vi "HardwareLoop.vi"(8 "Error In":errorcluster, 10 "Action Queues":T2, 11 "Executable Configuration":T1) -> (0 "Error Out":errorcluster)   [LabVIEW 2012]
uses:
  ActionQueues.ctl
  UIActionQueueElement.ctl
  UIAction.ctl
  HardwareActionQueueElement.ctl
  HardwareAction.ctl
  ExecutableConfiguration.ctl
  driver/Keithley-7001.lvlib
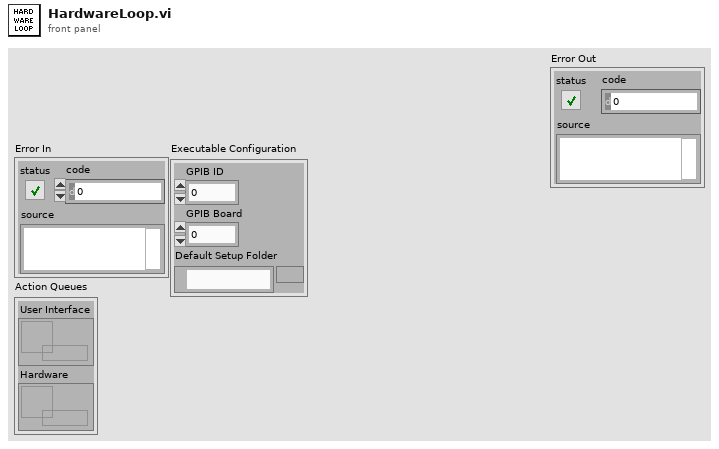
[diagram p1: front panel]
types:
  T1 = typedef "ExecutableConfiguration.ctl" = cluster{"GPIB ID":u8, "GPIB Board":u8, "Default Setup Folder":path}
  T2 = typedef "ActionQueues.ctl" = cluster{"User Interface":refnum<queue>, "Hardware":refnum<queue>}
  T3 = typedef "HardwareActionQueueElement.ctl" = cluster{"Action":T4, "Data":variant}
  T4 = typedef "HardwareAction.ctl" = enum16{"Initialize", "Start", "Stop", "Error", "Shutdown"}
  T5 = typedef "UIActionQueueElement.ctl" = cluster{"Action":T6, "Data":variant}
  T6 = typedef "UIAction.ctl" = enum16{"Initialize", "Configure Trigger", "Configure Scan", "Configure Memory", "Configure Slot 1", "Open", "Save", "Reset", "Start", "Started", "Stop", "Stopped", "Shutdown"}
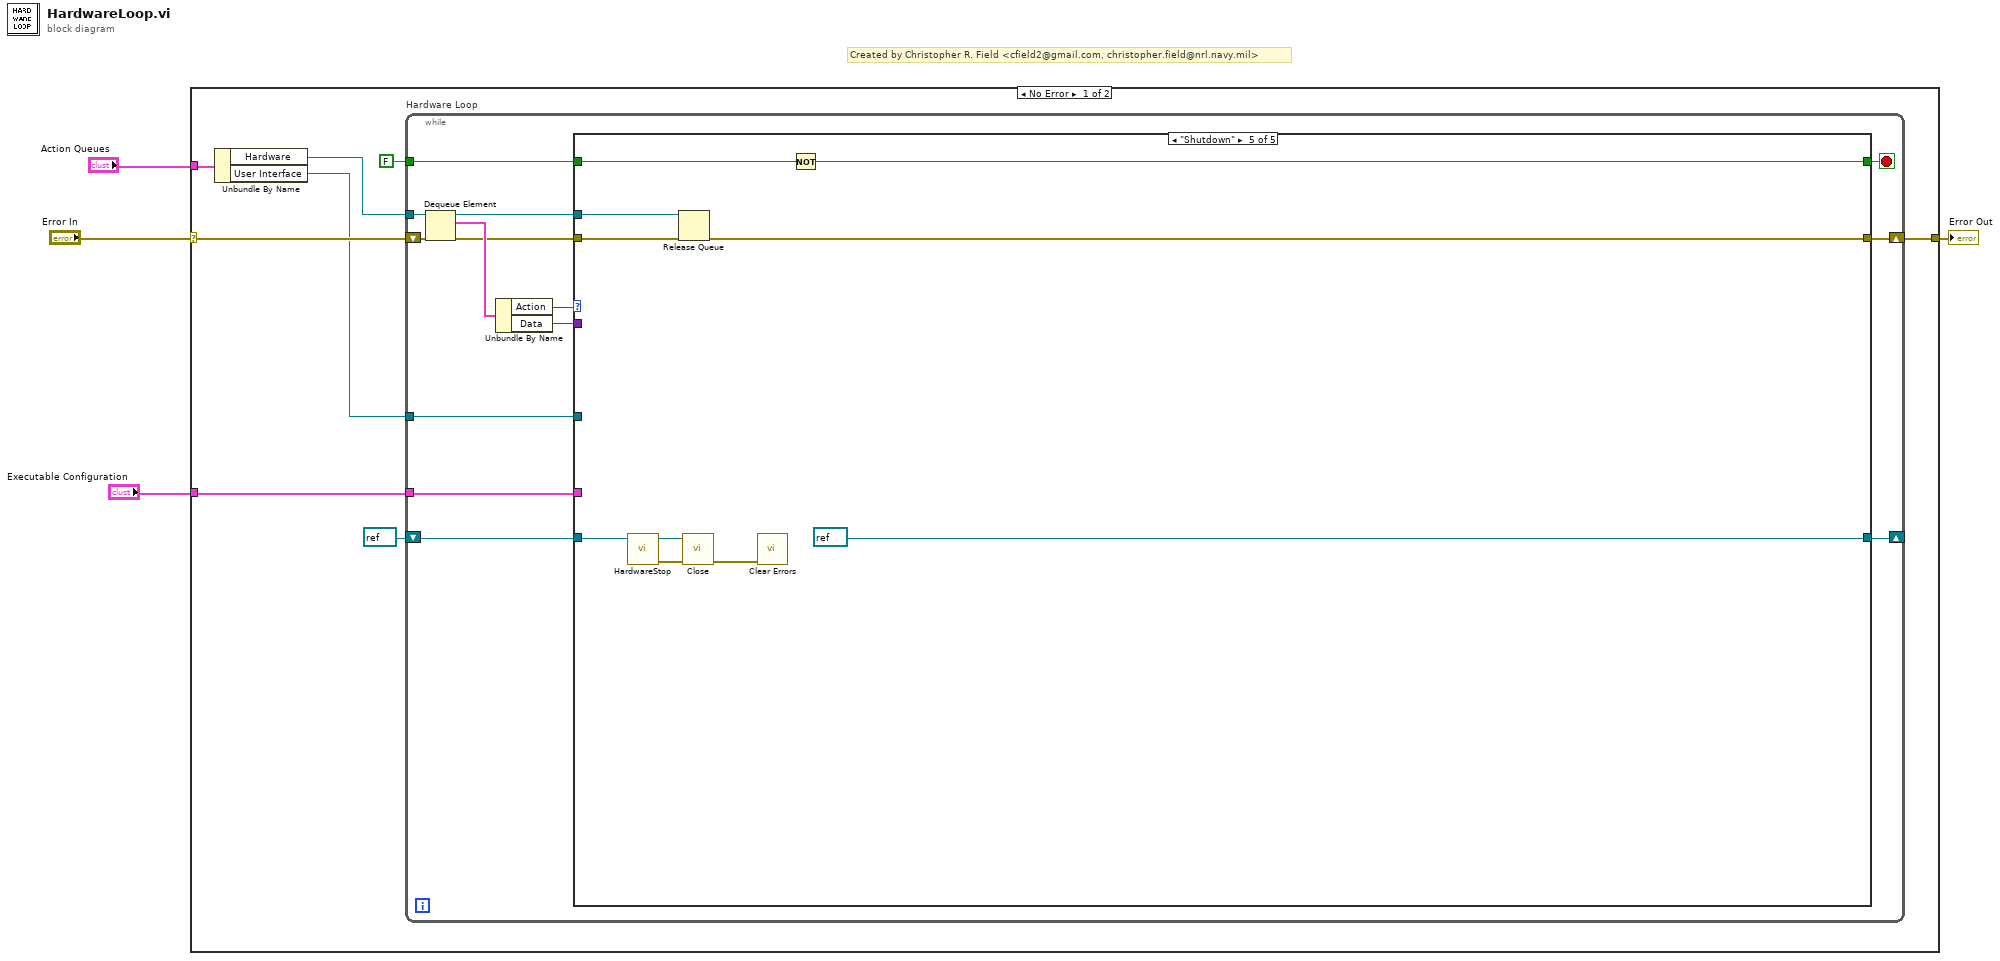
[diagram p0: block diagram]
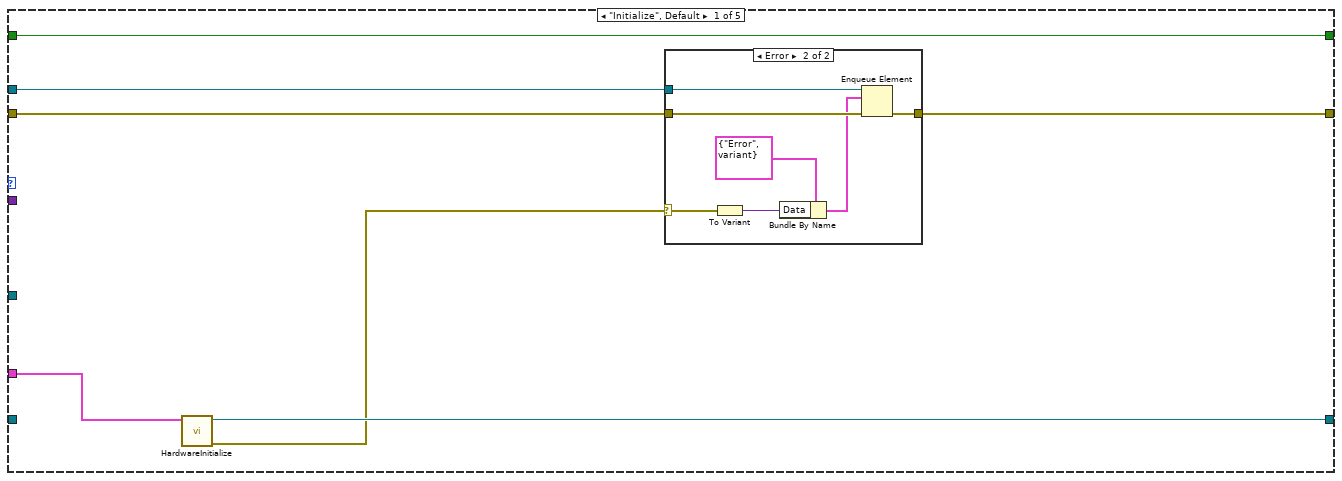
[diagram p2: hidden frame]
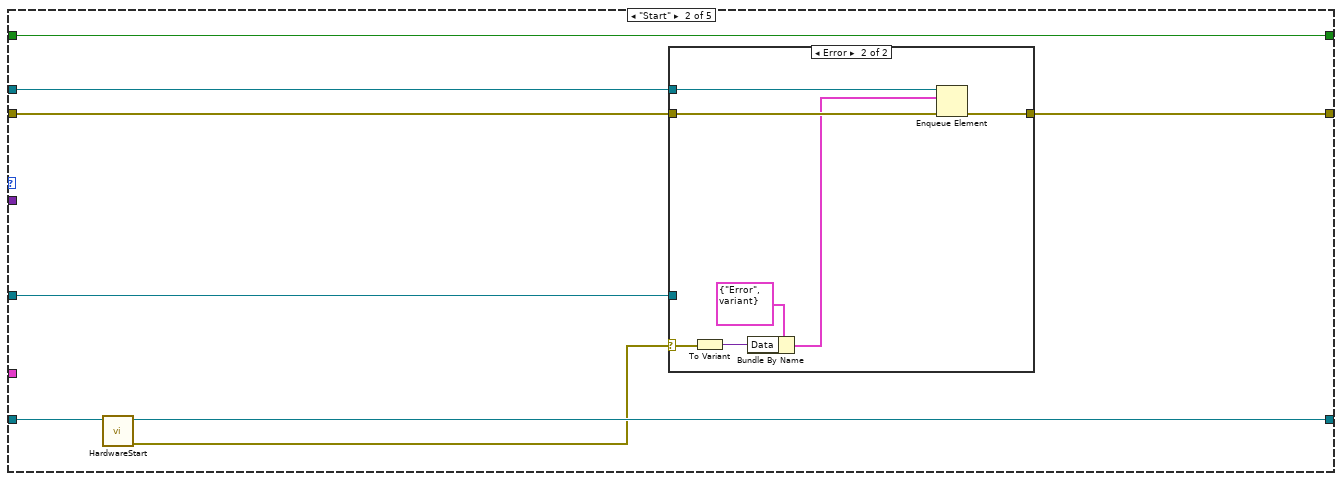
[diagram p4: hidden frame]
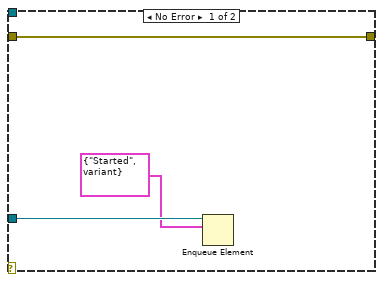
[diagram p5: hidden frame]
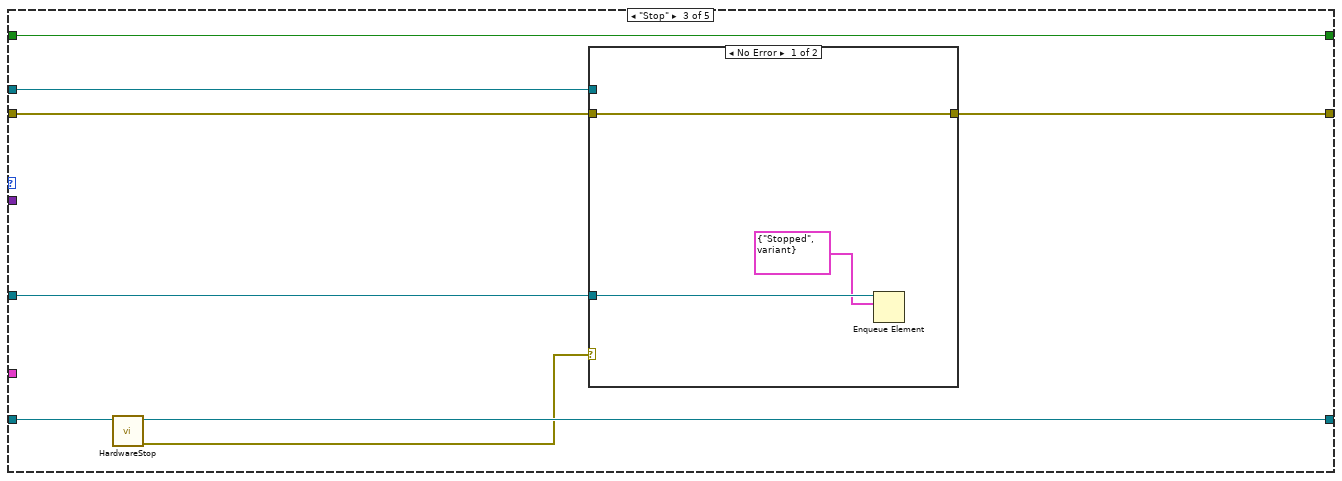
[diagram p6: hidden frame]
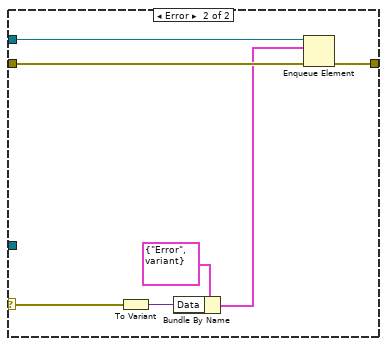
[diagram p7: hidden frame]
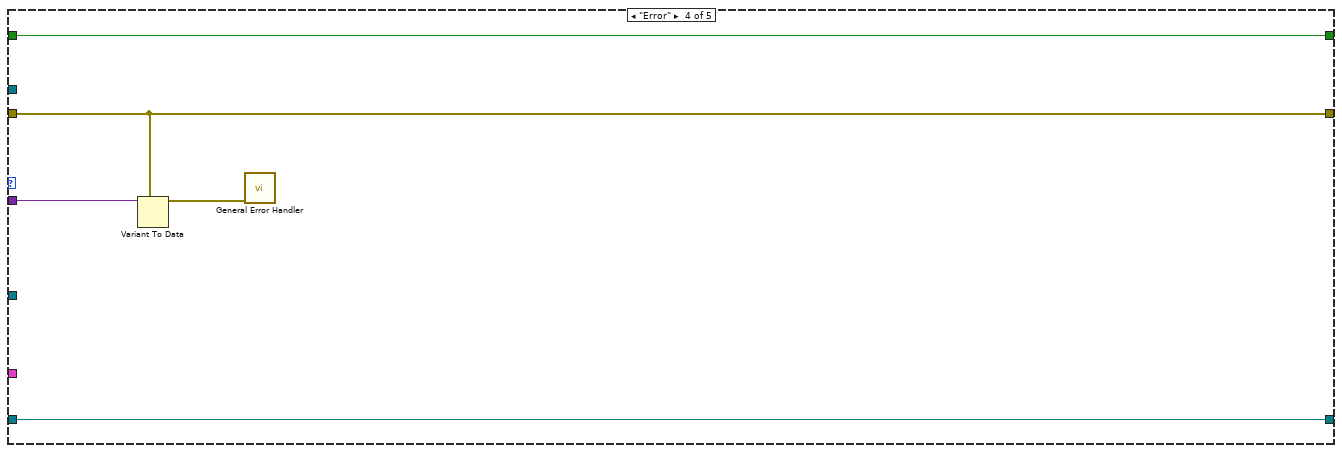
[diagram p8: hidden frame]
diagram:
  # "Created by Christopher R. Field <cfield2@gmail.com, christopher.field@nrl.navy.mil>"
  n1 = case shown="No Error" "Error In" {
    selector: "Error In" -> [w12 w93]
    tunnel: "Action Queues" -> [w11 _]
    tunnel: "Executable Configuration" -> [w7 _]
    tunnel: [w6 w93] -> w1
    frame No Error {
      n2 = Unbundle By Name(w11) -> ("Hardware"=w10:refnum<queue>, "User Interface"=w8:refnum<queue>)
      n3 = while "Hardware Loop" {
        tunnel: w10 -> [w25]
        shift-right: [w17] -> w6
        shift-left: w12 -> [w26]
        tunnel: FALSE -> [w19]
        tunnel: w8 -> [w16]
        tunnel: w7 -> [w15]
        shift-right: [w14] -> _
        shift-left: refnum<visa-resource-name> refnum ("Keithley 7001 Out") -> [w13]
        stop <- w18 stop-if-true
        n4 = Dequeue Element(queue=w25, error in (no error)=w26) -> (queue out=w20:refnum<queue>, element=w24:T3, error out=w21:errorcluster)  [unwired: 1 in, 1 out]
        n5 = Unbundle By Name(w24) -> ("Action"=w23:T4, "Data"=w22:variant)
        n6 = case shown="\"Shutdown\"" w23 {
          tunnel: w22 -> [_ _ _ w81 _]
          tunnel: w21 -> [w32 w44 w60 w80 w89]
          tunnel: w20 -> [w30 w45 w61 _ w90]
          tunnel: w19 -> [w33 w49 w67 w82 w92]
          tunnel: [w33 w49 w67 w82 w91] -> w18
          tunnel: [w31 w43 w64 w80 w88] -> w17
          tunnel: w16 -> [_ w42 w62 _ _]
          tunnel: w15 -> [w28 _ _ _ _]
          tunnel: [w29 w47 w65 w78 refnum<visa-resource-name> refnum ("Keithley 7001 Out")] -> w14
          tunnel: w13 -> [_ w48 w66 w78 w83]
          frame "Initialize", Default {
            n7 = call "HardwareInitialize.vi"("Executable Configuration"=w28) -> ("Error Out"=w27:errorcluster, "Keithley 7001 Out"=w29:refnum<visa-resource-name>)  [unwired: 9 in]
            n8 = case shown="Error" w27 {
              selector: w27 -> [_ w36]
              tunnel: w32 -> [w34 w41]
              tunnel: [w34 w40] -> w31
              tunnel: w30 -> [_ w39]
              frame No Error {
              }
              frame Error {
                n9 = To Variant(anything=w36) -> (Variant=w37:variant)
                n10 = Bundle By Name(cluster=T3 {"Action"=enum."Error", "Data"=variant} ("element"), "Data"=w37) -> (w35:T3)
                n11 = Enqueue Element(queue=w39, element=w35, error in (no error)=w41) -> (error out=w40:errorcluster)  [unwired: 1 in, 2 out]
              }
            }
          }
          frame "Start" {
            n12 = call "HardwareStart.vi"("Keithley 7001 In"=w48) -> ("Error Out"=w46:errorcluster, "Keithley 7001 Out"=w47:refnum<visa-resource-name>)  [unwired: 9 in]
            n13 = case shown="Error" w46 {
              selector: w46 -> [_ w54]
              tunnel: w45 -> [_ w59]
              tunnel: w44 -> [w52 w58]
              tunnel: [w52 w57] -> w43
              tunnel: w42 -> [w51 _]
              frame No Error {
                n14 = Enqueue Element(queue=w51, element=T5 {"Action"=enum."Started", "Data"=variant}) -> ()  [unwired: 2 in, 3 out]
              }
              frame Error {
                n15 = To Variant(anything=w54) -> (Variant=w55:variant)
                n16 = Bundle By Name(cluster=T3 {"Action"=enum."Error", "Data"=variant} ("element"), "Data"=w55) -> (w53:T3)
                n17 = Enqueue Element(queue=w59, element=w53, error in (no error)=w58) -> (error out=w57:errorcluster)  [unwired: 1 in, 2 out]
              }
            }
          }
          frame "Stop" {
            n18 = call "HardwareStop.vi"("Keithley 7001 In"=w66) -> ("Error Out"=w63:errorcluster, "Keithley 7001 Out"=w65:refnum<visa-resource-name>)  [unwired: 9 in]
            n19 = case shown="No Error" w63 {
              selector: w63 -> [_ w72]
              tunnel: w61 -> [_ w77]
              tunnel: w60 -> [w70 w76]
              tunnel: [w70 w75] -> w64
              tunnel: w62 -> [w69 _]
              frame No Error {
                n20 = Enqueue Element(queue=w69, element=T5 {"Action"=enum."Stopped", "Data"=variant}) -> ()  [unwired: 2 in, 3 out]
              }
              frame Error {
                n21 = To Variant(anything=w72) -> (Variant=w73:variant)
                n22 = Bundle By Name(cluster=T3 {"Action"=enum."Error", "Data"=variant} ("element"), "Data"=w73) -> (w71:T3)
                n23 = Enqueue Element(queue=w77, element=w71, error in (no error)=w76) -> (error out=w75:errorcluster)  [unwired: 1 in, 2 out]
              }
            }
          }
          frame "Error" {
            n24 = Variant To Data(type=w80, Variant=w81) -> (data=w79:errorcluster)  [unwired: 1 in, 1 out]
            n25 = call <vilib>:"General Error Handler.vi"("error in (no error)"=w79) -> ()  [unwired: 10 in, 5 out]
          }
          frame "Shutdown" {
            n26 = call "HardwareStop.vi"("Keithley 7001 In"=w83) -> ("Error Out"=w85:errorcluster, "Keithley 7001 Out"=w84:refnum<visa-resource-name>)  [unwired: 9 in]
            n27 = Release Queue(queue=w90, error in (no error)=w89) -> (error out=w88:errorcluster)  [unwired: 1 in, 2 out]
            n28 = call "Close.vi"("Error In"=w85, "Keithley 7001 In"=w84) -> ("Error Out"=w87:errorcluster)  [unwired: 9 in]
            n29 = call <vilib>:"Clear Errors.vi"("error in (no error)"=w87) -> ()  [unwired: 6 in, 1 out]
            n30 = Not(x=w92) -> (.not. x?=w91:bool)
          }
        }
      }
    }
    frame Error {
    }
  }
  "Error Out" <- w1
